vi "set replace existing.vi"(8 "error in (no error)":errorcluster, 10 "Replace existing":bool=TRUE, 11 "References":T1) -> (0 "error out":errorcluster, 3 "References out":T1)   [LabVIEW 2014, in "SQLite editor node.lvclass"]
uses:
  SQLite editor node.lvclass
  <vilib>/NI/DCAF/Tag Editor Core/Table API/Table Manager/object ref.ctl
  <vilib>/NI/DCAF/Tag Editor Core/Configuration Editor/Classes/Engine Parent/Engine Parent Editor Node.lvclass
  <vilib>/NI/DCAF/Tag Editor Core/Configuration Editor/Classes/Module editor node/module editor node.lvclass
  module/configuration/SQLite configuration.lvclass
  <vilib>/NI/Configuration Framework/serializable configuration/NISE_CEF_serializable configuration.lvclass
  <vilib>/NI/DCAF/Tag Editor Core/Table API/Table Manager/Table Manager.lvclass
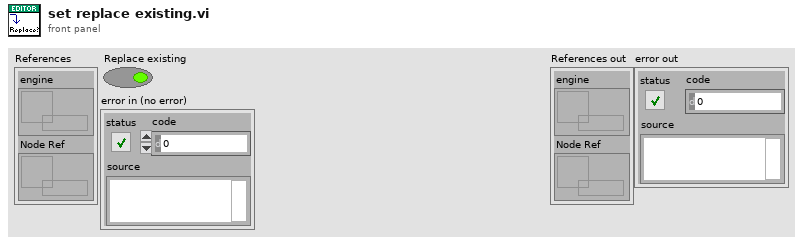
[diagram p1: front panel]
types:
  T1 = typedef "Table Manager.lvlib/Table Manager.lvclass/object ref.ctl" = cluster{"engine":refnum<data-value>, "Node Ref":refnum<data-value>}
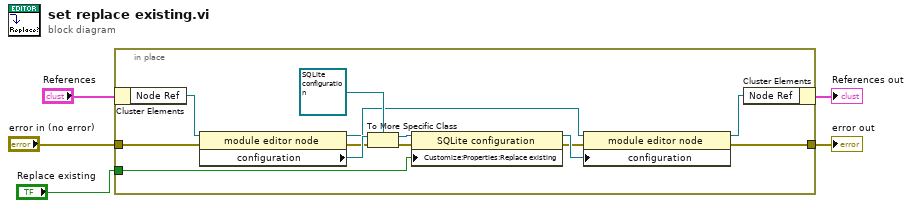
[diagram p0: block diagram]
diagram:
  n1 = in-place {
    in-place-border: "Replace existing" -> [w13]
    in-place-border: "error in (no error)" -> [w7]
    in-place-border: [w6] -> w1
    n2 = in-place-cluster #1("References") -> ("Node Ref"=w18:refnum<data-value>)
    n3 = property class="module editor node"(reference=w18, error in=w7) -> (reference out=w10:refnum<data-value>, error out=w15:errorcluster, "configuration"=w17:refnum<class "NISE_CEF_serializable configuration.lvclass">)
    n4 = To More Specific Class(target class=refnum<class "SQLite configuration.lvclass"> refnum ("SQLite configuration"), reference=w17, error in=w15) -> (specific class reference=w14:refnum<class "SQLite configuration.lvclass">, error out=w12:errorcluster)
    n5 = property class="SQLite configuration"(reference=w14, error in=w12, "Customize:Properties:Replace existing"=w13) -> (reference out=w11:refnum<class "SQLite configuration.lvclass">, error out=w9:errorcluster)
    n6 = property class="module editor node"(reference=w10, error in=w9, "configuration"=w11) -> (reference out=w8:refnum<data-value>, error out=w6:errorcluster)
    n7 = in-place-cluster #1("Node Ref"=w8) -> (→"References out":T1)
  }
  "error out" <- w1
